vi "LoadKeysFromFile.vi"(8 "error in (no error)":errorcluster, 11 "TrigBoxINIFileClass in":refnum<class "TrigBoxINIFileClass.lvclass">) -> (0 "error out":errorcluster, 3 "TrigBoxINIFileClass out":refnum<class "TrigBoxINIFileClass.lvclass">)   [LabVIEW 2013, in "TrigBoxINIFileClass.lvclass"]
uses:
  TrigBoxINIFileClass.lvclass
panel:
  out "RemoteAddress":string
  out "RemotePort":string
  out "LocalPort":string
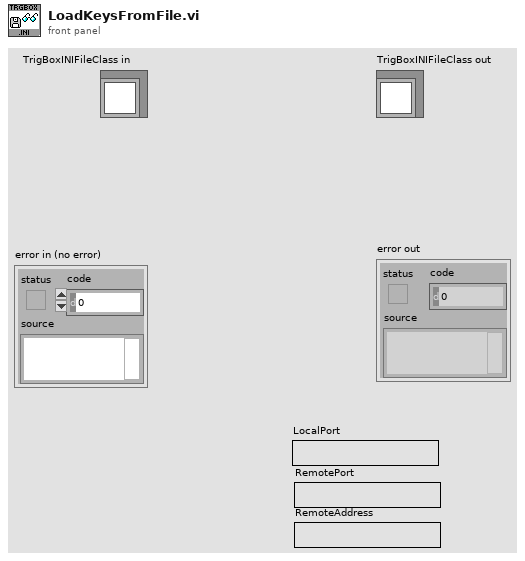
[diagram p1: front panel]
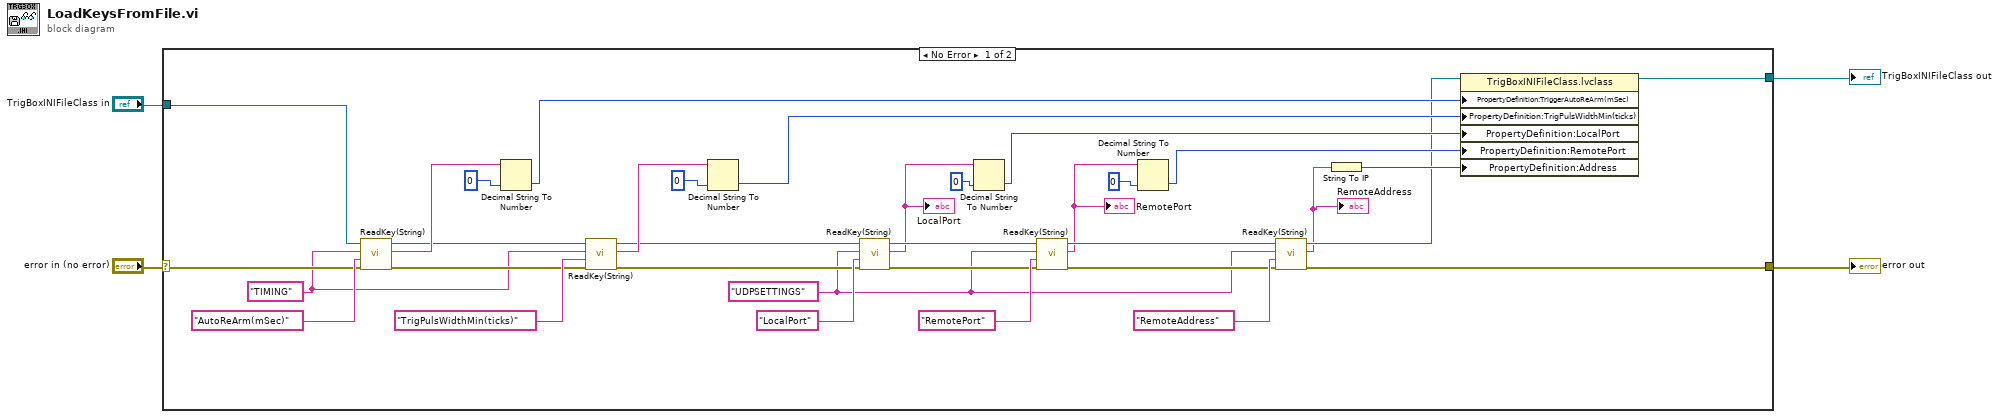
[diagram p0: block diagram]
diagram:
  n1 = case shown="No Error" "error in (no error)" {
    selector: "error in (no error)" -> [w12 w40]
    tunnel: [w23 w40] -> w3
    tunnel: [w9 w39] -> w1
    tunnel: "TrigBoxINIFileClass in" -> [w19 w39]
    frame No Error {
      w20 = "UDPSETTINGS" ("section")
      w10 = "TIMING" ("section")
      n2 = call-dynamic "ReadKey(String).vi"("error in"=w12, "key"="AutoReArm(mSec)" ("section"), "section"=w10, "INIFileClass in"=w19) -> ("error out"=w11:errorcluster, "StringOut"=w36:string, "INIFileClass out"=w33:refnum<class "TrigBoxINIFileClass.lvclass">)  [unwired: 5 in]
      n3 = Decimal String To Number(string=w36, default (0L)=i64 0) -> (number=w14:i64)  [unwired: 1 in, 1 out]
      n4 = call-dynamic "ReadKey(String).vi"("error in"=w11, "key"="TrigPulsWidthMin(ticks)", "section"=w10, "INIFileClass in"=w33) -> ("error out"=w21:errorcluster, "StringOut"=w34:string, "INIFileClass out"=w22:refnum<class "TrigBoxINIFileClass.lvclass">)  [unwired: 5 in]
      n5 = Decimal String To Number(string=w34, default (0L)=u64 0) -> (number=w13:u64)  [unwired: 1 in, 1 out]
      n6 = call-dynamic "ReadKey(String).vi"("error in"=w21, "key"="LocalPort" ("section"), "section"=w20, "INIFileClass in"=w22) -> ("error out"=w28:errorcluster, "StringOut"=w7:string, "INIFileClass out"=w27:refnum<class "TrigBoxINIFileClass.lvclass">)  [unwired: 5 in]
      "LocalPort" <- w7
      n7 = Decimal String To Number(string=w7, default (0L)=u16 0 ("default (0 I32)")) -> (number=w15:u16)  [unwired: 1 in, 1 out]
      n8 = call-dynamic "ReadKey(String).vi"("error in"=w28, "key"="RemotePort" ("section"), "section"=w20, "INIFileClass in"=w27) -> ("error out"=w24:errorcluster, "StringOut"=w6:string, "INIFileClass out"=w25:refnum<class "TrigBoxINIFileClass.lvclass">)  [unwired: 5 in]
      "RemotePort" <- w6
      n9 = Decimal String To Number(string=w6, default (0L)=u16 0 ("default (0 I32)")) -> (number=w17:u16)  [unwired: 1 in, 1 out]
      n10 = call-dynamic "ReadKey(String).vi"("error in"=w24, "key"="RemoteAddress" ("section"), "section"=w20, "INIFileClass in"=w25) -> ("error out"=w23:errorcluster, "StringOut"=w5:string, "INIFileClass out"=w8:refnum<class "TrigBoxINIFileClass.lvclass">)  [unwired: 5 in]
      "RemoteAddress" <- w5
      n11 = String To IP(1:w5) -> (0:w16:u32)
      n12 = property class="TrigBoxINIFileClass.lvclass"(reference=w8, "PropertyDefinition:TriggerAutoReArm(mSec)"=w14, "PropertyDefinition:TrigPulsWidthMin(ticks)"=w13, "PropertyDefinition:LocalPort"=w15, "PropertyDefinition:RemotePort"=w17, "PropertyDefinition:Address"=w16) -> (reference out=w9:refnum<class "TrigBoxINIFileClass.lvclass">)  [unwired: 1 in, 1 out]
    }
    frame Error {
    }
  }
  "error out" <- w3
  "TrigBoxINIFileClass out" <- w1
